vi "Draw Rect Direct FIFO 100.vi"(8 "error in (no error)":errorcluster, 9 "Cluster":T1, 11 "Refnum in":refnum<k20>) -> (0 "error out":errorcluster, 3 "Refnum out":refnum<k20>)   [LabVIEW 2013]
uses:
  Cluser.ctl
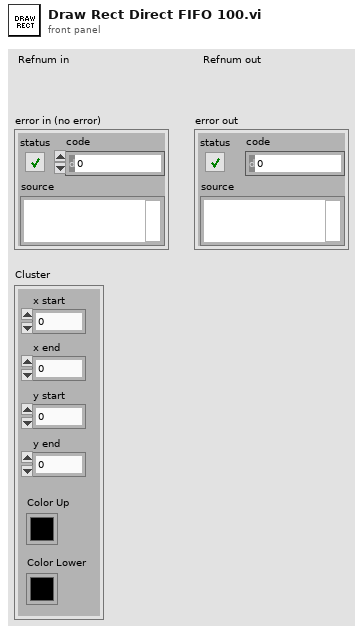
[diagram p1: front panel]
types:
  T1 = typedef "Cluser.ctl" = cluster{"x start":u16, "x end":u16, "y start":u16, "y end":u16, "Color Up":u32, "Color Lower":u32}
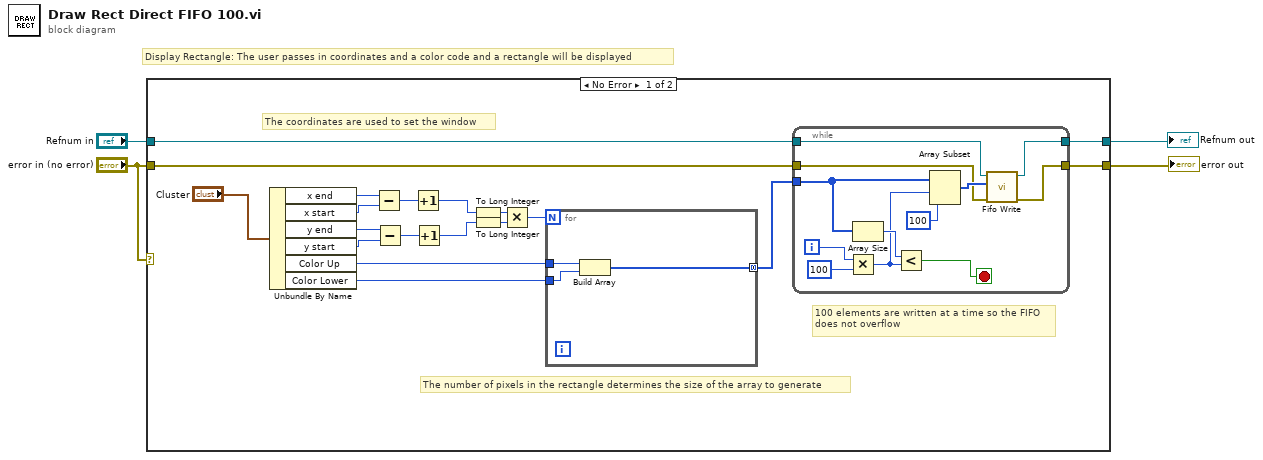
[diagram p0: block diagram]
diagram:
  # "Display Rectangle: The user passes in coordinates and a color code and a rectangle will be displayed"
  n1 = case shown="No Error" "error in (no error)" {
    tunnel: "error in (no error)" -> [w5 w39]
    tunnel: "Refnum in" -> [w6 w40]
    tunnel: [w7 w40] -> w1
    tunnel: [w8 w39] -> w3
    frame No Error {
      # "100 elements are written at a time so the FIFO\ndoes not overflow"
      # "The number of pixels in the rectangle determines the size of the array to generate"
      # "The coordinates are used to set the window"
      n2 = Unbundle By Name("Cluster") -> ("x end"=w22:u16, "x start"=w21:u16, "y end"=w20:u16, "y start"=w19:u16, "Color Up"=w14:u32, "Color Lower"=w13:u32)
      n3 = Subtract(x=w22, y=w21) -> (x-y=w18:u16)
      n4 = Subtract(x=w20, y=w19) -> (x-y=w17:u16)
      n5 = Increment(x=w18) -> (x+1=w12:u16)
      n6 = Increment(x=w17) -> (x+1=w11:u16)
      n7 = To Long Integer(number=w12) -> (32bit integer=w16:i32)
      n8 = To Long Integer(number=w11) -> (32bit integer=w15:i32)
      n9 = Multiply(x=w16, y=w15) -> (x*y=w10:i32)
      n10 = for {
        N: w10 -> [_]
        tunnel: w14 -> [w38]
        tunnel: w13 -> [w37]
        tunnel: [w36] -> w9 mode=concatenating
        n11 = Build Array(w38, w37) -> (w36:u32[])
      }
      n12 = while {
        tunnel: w9 -> [w31]
        tunnel: w6 -> [w24]
        tunnel: w5 -> [w27]
        tunnel: [w26] -> w8
        tunnel: [w25] -> w7
        i -> [w34]
        stop <- w30 stop-if-true
        n13 = Multiply(x=w34, y=100) -> (x*y=w29:i32)
        n14 = Array Size(array=w31) -> (size(s)=w32:i32)
        n15 = Less?(x=w32, y=w29) -> (x < y?=w30:bool)
        n16 = Array Subset(array=w31, index=w29, length=100) -> (w28:u32[])
        n17 = call "Fifo Write.vi"("error in (no error)"=w27, "Data"=w28, "Refnum in"=w24) -> ("error out"=w26:errorcluster, "Refnum out"=w25:refnum<k20>)  [unwired: 7 in]
      }
    }
    frame Error {
    }
  }
  "error out" <- w3
  "Refnum out" <- w1
